vi "LSX Set Analog Output.vi"(8 "error in (no error)":errorcluster, 9 "lValue":i32, 10 "lIndex":i32, 11 "lLSID":i32) -> (0 "error out":errorcluster, 3 "function return":i32)   [LabVIEW 2018, in "Tango.lvlib"]
doc: "TANGOAPI int TANGOCALL LSX_SetAnalogOutput (int lLSID, int lIndex, int lValue);"
uses:
  Tango.lvlib
  SubVIs/Tango_DLL.dll
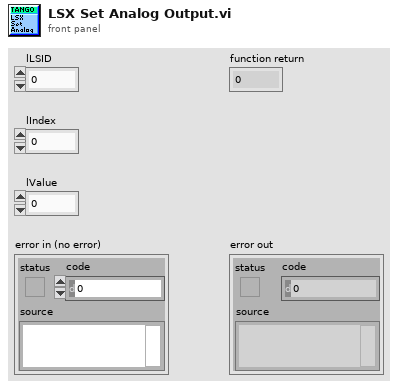
[diagram p1: front panel]
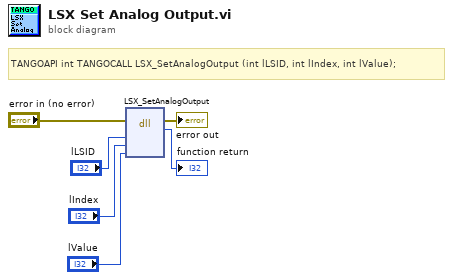
[diagram p0: block diagram]
diagram:
  # "TANGOAPI int TANGOCALL LSX_SetAnalogOutput (int lLSID, int lIndex, int lValue);"
  n1 = dll-call lib="C:/Users/Familie/Documents/LabviewIX81/lib/TANGO Stage/SubVIs/Tango_DLL.*" fn="LSX_SetAnalogOutput"(error in="error in (no error)", "lLSID"="lLSID", "lIndex"="lIndex", "lValue"="lValue") -> (error out=→"error out":errorcluster, →"function return":i32)  [unwired: 5 in, 1 out]
